vi "DSF.Shared.Configuration.Transfer Group.Create From String.vi"(8 "error in (no error)":errorcluster, 10 "String":string) -> (0 "error out":errorcluster, 3 "Transfer Group Configuration out":refnum<class "DSF.Shared.Configuration.Transfer Group.lvclass">)   [LabVIEW 2016, in "DSF.Shared.lvlib" / "DSF.Shared.Configuration.Transfer Group.lvclass"]
uses:
  DSF.Shared.Configuration.Transfer Group.lvclass
  C:/Git/Sourcetree/DSF/Source/Shared/Classes/Configuration/DSF.Shared.Configuration.lvclass
  Configuration/DSF.Shared.Configuration.lvclass
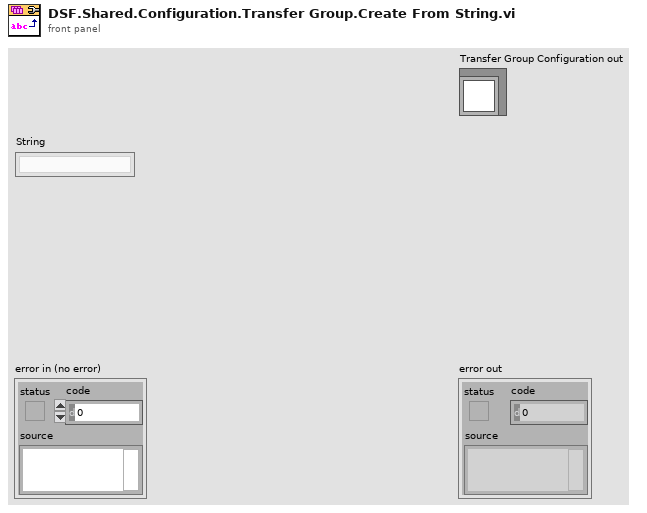
[diagram p1: front panel]
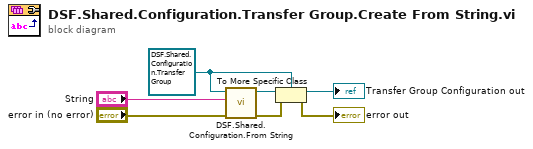
[diagram p0: block diagram]
diagram:
  w6 = refnum<class "DSF.Shared.Configuration.Transfer Group.lvclass"> refnum ("Transfer Configuration out")
  n1 = call "DSF.Shared.Configuration.From String.vi"("error in (no error)"="error in (no error)", "String"="String", "Configuration in"=w6) -> ("error out"=w3:errorcluster, "Configuration out"=w7:refnum<class "DSF.Shared.Configuration.lvclass">)  [unwired: 7 in]
  n2 = To More Specific Class(target class=w6, reference=w7, error in=w3) -> (specific class reference=→"Transfer Group Configuration out":refnum<class "DSF.Shared.Configuration.Transfer Group.lvclass">, error out=→"error out":errorcluster)
